vi "AlliGator Save Raw Phasor v2.vi"(4 "Save only if selected":bool, 6 "Save as...":bool, 7 "Phasor Plot Path (empty)":path, 8 "error in (no error)":errorcluster, 9 "Raw Phasor Plot":T1={"Phasor Plot Name"="", "Raw Phasor Plot"=[], "Phasor Frequency"=160000000.0, "[Decay Metadata]"=[], "Raw Phasor Plot SDV"=[], "Phasor SDV Options"={"Compute Estimated SDV"=FALSE, "# Replicas"=100, "Use Estimated Average Phasor"=FALSE}, "[Calibration Phasor]"=[]} {"[Decay Metadata]"."# Folds" min=1; "[Decay Metadata]"."ROI Descriptor"."Contours"."Type" items=["No Selection", "Point", "Line", "Rectangle", "Oval", "Polygon", "Freehand Region", "Annulus", "Unused2", "Unused3", "Broken Line", "Freehand Line", "Rotated Rectangle"]}, 10 "Selected Plot":i32, 11 "Phasor Graph":refnum<vi>) -> (0 "Error Out":errorcluster, 2 "Message":string)   [LabVIEW 2021, in "AlliGator Phasor Graph.lvlib"]
doc: "Saves raw phasor plot data and associated data and metadata to .phplot file."
uses:
  AlliGator Phasor Graph.lvlib
  AlliGator Raw Phasor Plot Data v4.ctl
  Phasor/Phasor (g, s).ctl
  AlliGator Decay Metadata v3.ctl
  AlliGator Decay Background Subtraction Info.ctl
  AlliGator Baseline Subtraction Method.ctl
  Graphs/XY Graph/XY Graph Plot Shift Parameters.ctl
  Graphs/XY Graph/XY Graph Plot Shift Method.ctl
  AlliGator Decay Extrapolation Parameters.ctl
  Phasor/Phasor Standard Deviation Options.ctl
  Phasor/Calibration Phasor (m, phi).ctl
  75e45e5e-2a8e-42f3-a5de-cf34ebc50bf0.vi
  <vilib>/JDP Science/JSONtext/Variant to JSON Text.vi
  <vilib>/JDP Science/JSONtext/LVClass Serializer/JSONtext LVClass Serializer.lvclass
  Phasor/Phasor.lvlib
  AlliGator Decay Preprocessing.lvlib
  Graphs/XY Graph/XY Graph Add-Ons.lvlib
panel:
  # "see the AlliGator License on the block diagram (Ctrl+E or Window:Show Block Diagram)"
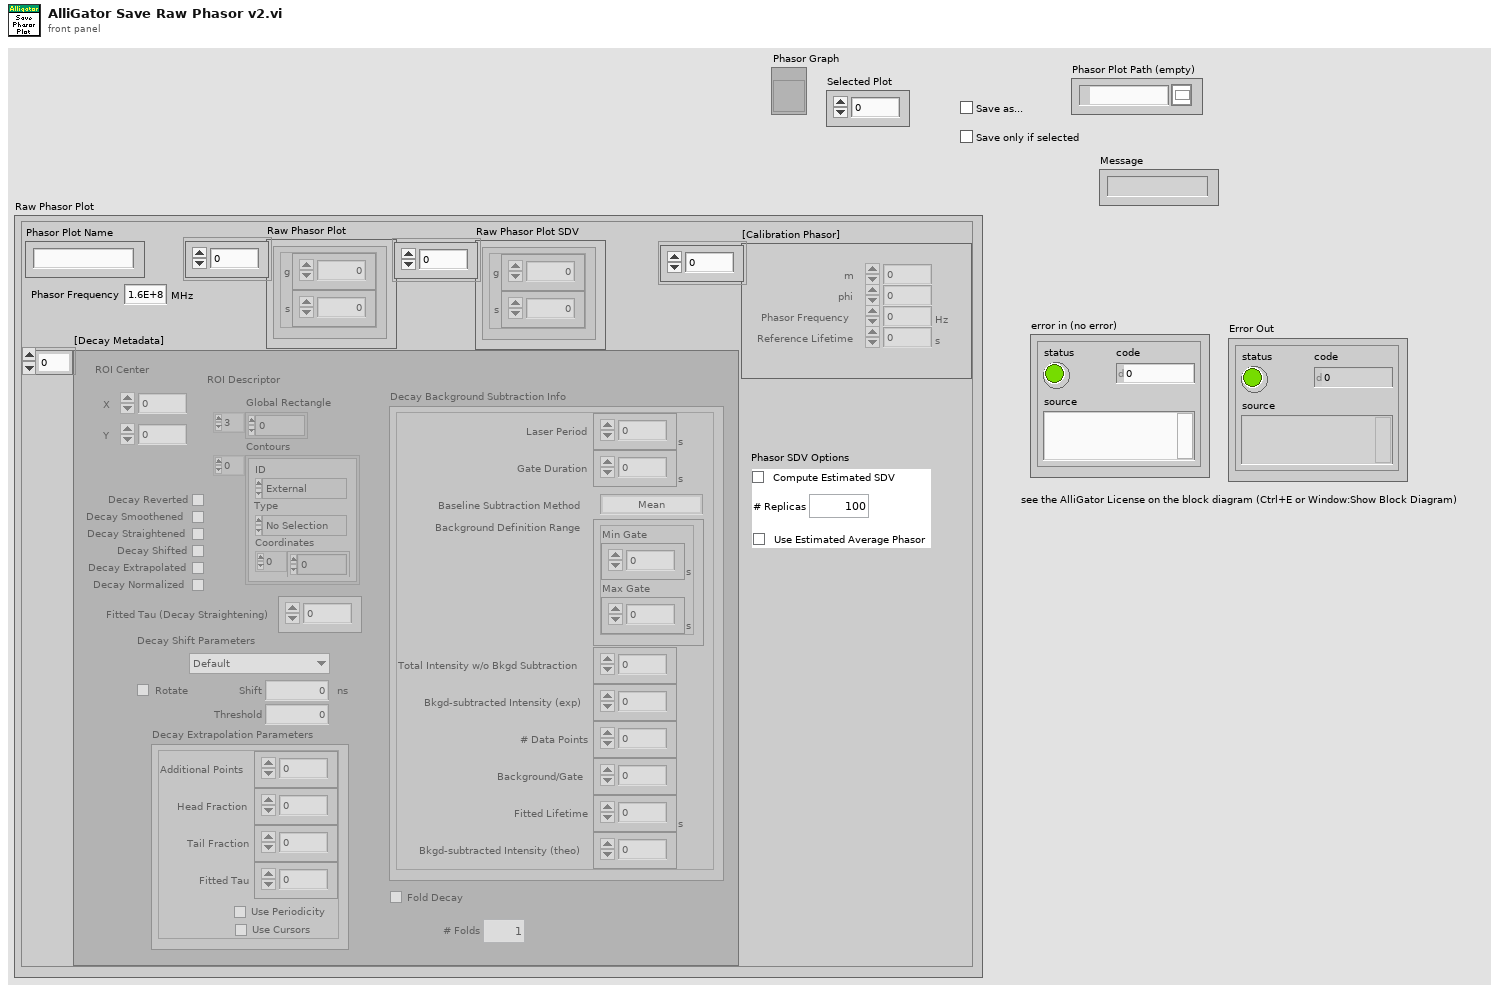
[diagram p1: front panel]
types:
  T1 = typedef "AlliGator Phasor Graph.lvlib/AlliGator Raw Phasor Plot Data v4.ctl" = cluster{"Phasor Plot Name":string, "Raw Phasor Plot":T2[], "Phasor Frequency":dbl[unit], "[Decay Metadata]":T3[], "Raw Phasor Plot SDV":T2[], "Phasor SDV Options":T10, "[Calibration Phasor]":T11[]}
  T2 = typedef "Phasor.lvlib/Phasor (g, s).ctl" = cluster{"g":dbl, "s":dbl}
  T3 = typedef "AlliGator Phasor Graph.lvlib/AlliGator Decay Metadata v3.ctl" = cluster{"ROI Descriptor":T4, "ROI Center":cluster{"X":i32, "Y":i32}, "Decay Background Subtraction Info":T5, "Decay Reverted":bool, "Decay Smoothened":bool, "Decay Straightened":bool, "Fitted Tau (Decay Straightening)":dbl, "Decay Shift Parameters":T7, "Decay Shifted":bool, "Decay Extrapolated":bool, "Decay Extrapolation Parameters":T9, "Decay Normalized":bool, "Fold Decay":bool, "# Folds":u32}
  T4 = typedef "ROI Descriptor" = cluster{"Global Rectangle":i32[], "Contours":cluster{"ID":enum32{"External", "Internal"}, "Type":u32, "Coordinates":i32[]}[]}
  T5 = typedef "AlliGator Decay Analysis.lvlib/AlliGator Decay Preprocessing.lvlib/AlliGator Decay Background Subtraction Info.ctl" = cluster{"Laser Period":dbl[unit], "Gate Duration":dbl[unit], "Baseline Subtraction Method":T6, "Background Definition Range":cluster{"Min Gate":dbl[unit], "Max Gate":dbl[unit]}, "Total Intensity w/o Bkgd Subtraction":dbl, "Bkgd-subtracted Intensity (exp)":dbl, "# Data Points":i32, "Background/Gate":dbl, "Fitted Lifetime":dbl[unit], "Bkgd-subtracted Intensity (theo)":dbl}
  T6 = typedef "AlliGator Decay Analysis.lvlib/AlliGator Decay Preprocessing.lvlib/AlliGator Baseline Subtraction Method.ctl" = enum16{"Mean", "Min", "Square Gated Single-Exponential", "File", "Constant"}
  T7 = typedef "XY Graph Add-Ons.lvlib/XY Graph Plot Shift Parameters.ctl" = cluster{"Type":T8, "Shift":dbl[unit], "Threshold":dbl, "Rotate":bool}
  T8 = typedef "XY Graph Add-Ons.lvlib/XY Graph Plot Shift Method.ctl" = enum16{"Default", "CFD", "Threshold", "Cross-Correlation"}
  T9 = typedef "AlliGator Decay Analysis.lvlib/AlliGator Decay Preprocessing.lvlib/AlliGator Decay Extrapolation Parameters.ctl" = cluster{"Additional Points":u32, "Head Fraction":dbl, "Fitted Tau":dbl, "Use Periodicity":bool, "Use Cursors":bool, "Tail Fraction":dbl}
  T10 = typedef "Phasor.lvlib/Phasor Standard Deviation Options.ctl" = cluster{"Compute Estimated SDV":bool, "# Replicas":u32, "Use Estimated Average Phasor":bool}
  T11 = typedef "Phasor.lvlib/Calibration Phasor (m, phi).ctl" = cluster{"m":dbl, "phi":dbl, "Phasor Frequency":dbl[unit], "Reference Lifetime":dbl[unit]}
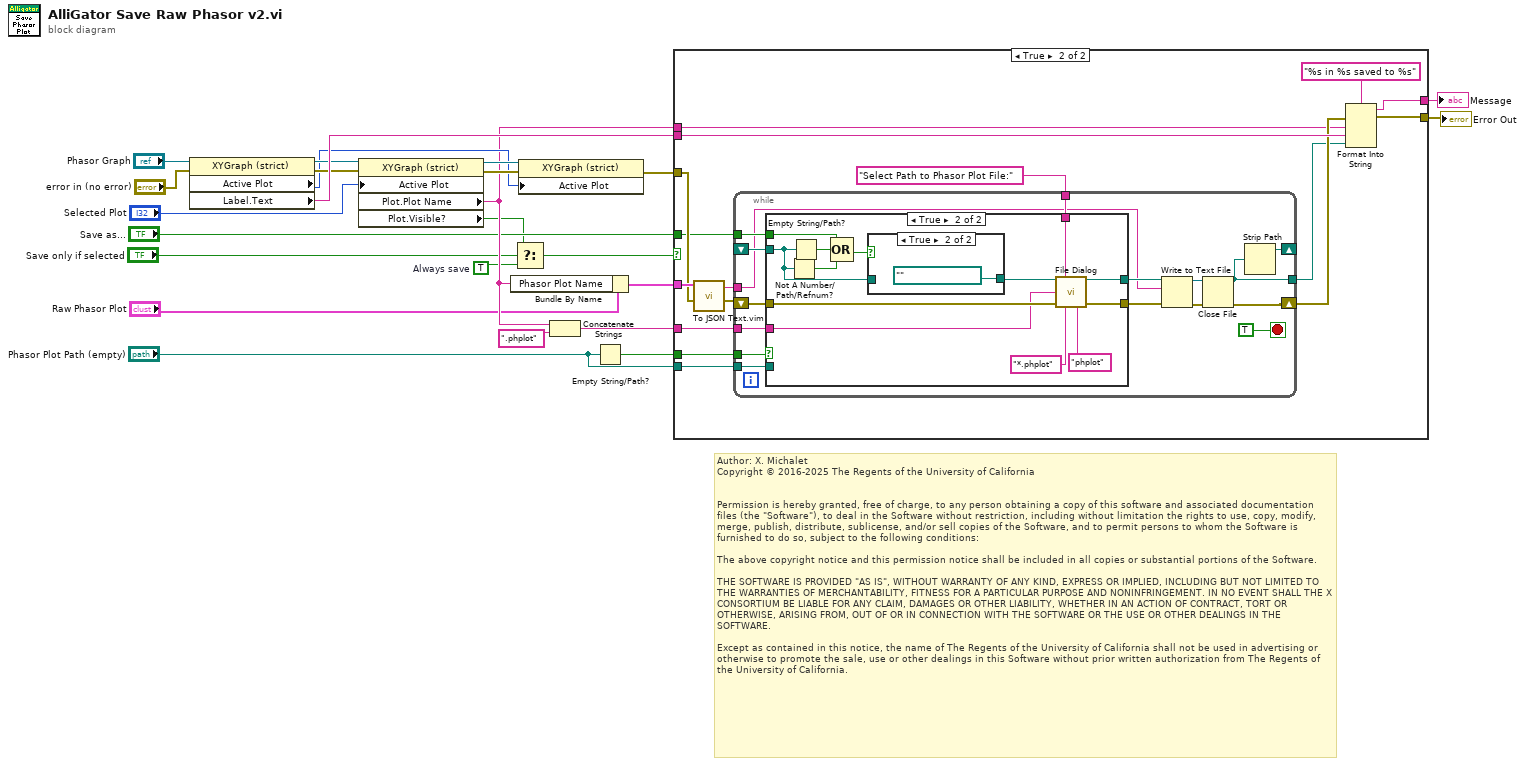
[diagram p0: block diagram]
diagram:
  w4 = TRUE  # Always save
  # "Author: X. Michalet\nCopyright © 2016-2025 The Regents of the University of California\n \n\nPermission is hereby granted, free of charge, to any person obtaining a copy of this software and associated documentation files (the \"Software\"), to deal in the Software without restriction, including without limitation the rights to use, copy, modify, merge, publish, distribute, sublicense, and/or sell copies of the Software, and to permit persons to whom the Software is furnished to do so, subject to the following conditions:\n\nThe above copyright notice and this permission notice shall be included in all copies or substantial portions of the Software.\n\nTHE SOFTWARE IS PROVIDED \"AS IS\", WITHOUT WARRANTY OF ANY KIND, EXPRESS OR IMPLIED, INCLUDING BUT NOT LIMITED TO THE WARRANTIES OF MERCHANTABILITY, FITNESS FOR A PARTICULAR PURPOSE AND NONINFRINGEMENT. IN NO EVENT SHALL THE X CONSORTIUM BE LIABLE FOR ANY CLAIM, DAMAGES OR OTHER LIABILITY, WHETHER IN AN ACTION OF CONTRACT, TORT OR OTHERWISE, ARISING FROM, OUT OF OR IN CONNECTION WITH THE SOFTWARE OR THE USE OR OTHER DEALINGS IN THE SOFTWARE.\n\nExcept as contained in this notice, the name of The Regents of the University of California shall not be used in advertising or otherwise to promote the sale, use or other dealings in this Software without prior written authorization from The Regents of the University of California."
  n1 = property class="XYGraph (strict)"(reference="Phasor Graph", error in="error in (no error)") -> (reference out=w20:refnum<vi>, error out=w19:errorcluster, "Active Plot"=w16:u32, "Label.Text"=w23:string)
  n2 = property class="XYGraph (strict)"(reference=w20, error in=w19, "Active Plot"="Selected Plot") -> (reference out=w18:refnum<vi>, error out=w17:errorcluster, "Plot.Plot Name"=w14:string, "Plot.Visible?"=w3:bool)
  n3 = Bundle By Name(cluster="Raw Phasor Plot", "Phasor Plot Name"=w14) -> (w10:T1)
  n4 = Select(t=w3, s="Save only if selected", f=w4) -> (s? t:f=w2:bool)
  n5 = property class="XYGraph (strict)"(reference=w18, error in=w17, "Active Plot"=w16) -> (error out=w9:errorcluster)  [unwired: 1 out]
  n6 = Concatenate Strings(w14, ".phplot" ("string")) -> (w11:string)
  n7 = Empty String/Path?(string/path="Phasor Plot Path (empty)") -> (empty?=w7:bool)
  n8 = case shown="True" w2 {
    tunnel: w23 -> [_ w40]
    tunnel: [w25 w26] -> w15
    tunnel: w14 -> [_ w37]
    tunnel: w11 -> [_ w35]
    tunnel: w10 -> [_ w34]
    tunnel: w9 -> [w25 w32]
    tunnel: "Save as..." -> [_ w30]
    tunnel: w7 -> [_ w29]
    tunnel: "Phasor Plot Path (empty)" -> [_ w28]
    tunnel: [_ w27] -> w1
    frame False {
    }
    frame True {
      n9 = call "To JSON Text.vim"("error in (no error)"=w32, "Anything"=w34) -> ("error out"=w31:errorcluster, "<JSON>"=w33:string)  [unwired: 8 in]
      n10 = while {
        tunnel: w33 -> [w48]
        tunnel: [w44] -> w38
        shift-right: [w45] -> w39
        shift-left: w31 -> [w52]
        shift-right: [w57] -> _
        shift-left: _ -> [w54]
        tunnel: w30 -> [w55]
        tunnel: "Select Path to Phasor Plot File:" ("Prompt") -> [w53]
        tunnel: w35 -> [w51]
        tunnel: w29 -> [w43]
        tunnel: w28 -> [w42]
        stop <- TRUE stop-if-true
        n11 = case shown="True" w43 {
          tunnel: w55 -> [_ w70]
          tunnel: w54 -> [_ w68]
          tunnel: w53 -> [_ w66]
          tunnel: w52 -> [w58 w65]
          tunnel: w51 -> [_ w62]
          tunnel: [w59 w61] -> w50
          tunnel: [w58 w60] -> w49
          tunnel: w42 -> [w59 _]
          frame False {
          }
          frame True {
            n12 = Not A Number/Path/Refnum?(number/path/refnum=w68) -> (NaN/Path/Refnum?=w71:bool)
            n13 = Empty String/Path?(string/path=w68) -> (empty?=w72:bool)
            n14 = Compound Arithmetic op=OR(w70, w72, w71) -> (w69:bool)
            n15 = case shown="True" w69 {
              tunnel: [w73 path "" ("start path  (Not A Path)")] -> w67
              tunnel: w68 -> [w73 _]
              frame False {
              }
              frame True {
              }
            }
            n16 = call "File Dialog"("start path"=w67, "prompt"=w66, "default name"=w62, "error in"=w65, "pattern (all files)"="*.phplot" ("Pattern (*.xml;*.XML)"), "pattern label"="phplot" ("File Extension (xml)")) -> ("selected path"=w61:path, "error out"=w60:errorcluster)  [unwired: 6 in, 2 out]
          }
        }
        n17 = Write to Text File(file (use dialog)=w50, text=w48, error in=w49) -> (refnum out=w47:refnum<file>, error out=w46:errorcluster)  [unwired: 1 in, 1 out]
        n18 = Close File(refnum=w47, error in=w46) -> (path=w44:path, error out=w45:errorcluster)
        n19 = Strip Path(path=w44) -> (stripped path=w57:path)  [unwired: 1 out]
      }
      n20 = Format Into String(format string="%s in %s saved to %s", error in=w39, w37, w40, w38) -> (resulting string=w27:string, error out=w26:errorcluster)  [unwired: 1 in]
    }
  }
  "Error Out" <- w15
  "Message" <- w1
